vi "Two While Loops.vi"() -> ()   [LabVIEW 2014]
panel:
  out "Bot Variable Stop":bool
  out "Top Variable Stop":bool
  out "Bottom Count":dbl
  in  "stop":bool
  out "Top Count":dbl
  # "Two While Loops"
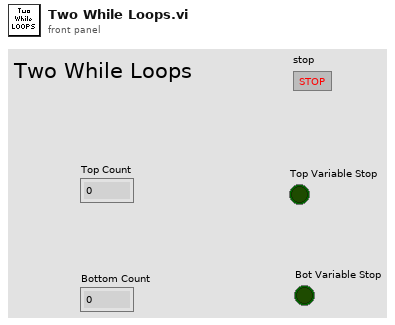
[diagram p1: front panel]
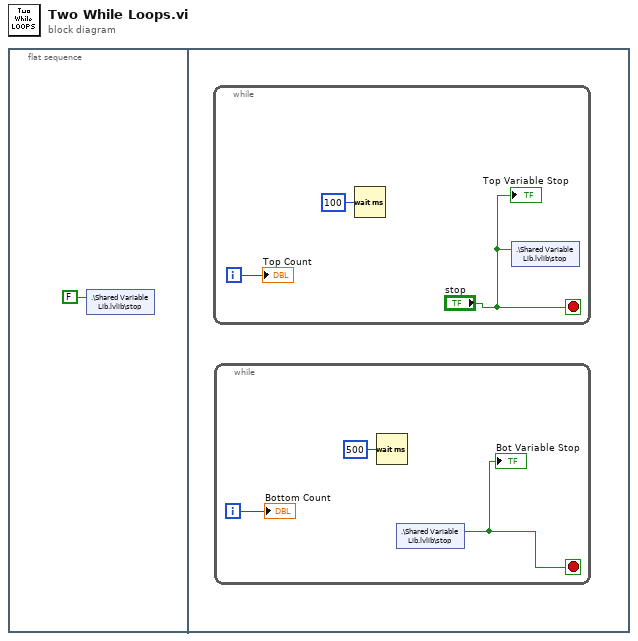
[diagram p0: block diagram]
diagram:
  n1 = flat-sequence {
    frame #0 {
      n2 = shared-variable ".\\Shared Variable Lib.lvlib\\stop"(FALSE ("stop")) -> ()  [unwired: 1 in, 1 out]
    }
    frame #1 {
      n3 = while {
        i -> [w6]
        stop <- "stop" stop-if-true
        n4 = Wait (ms)(milliseconds to wait=u32 100) -> ()  [unwired: 1 out]
        n5 = shared-variable ".\\Shared Variable Lib.lvlib\\stop"("stop") -> ()  [unwired: 1 in, 1 out]
        "Top Count" <- w6
        "Top Variable Stop" <- "stop"
      }
      n6 = while {
        i -> [w4]
        stop <- w2 stop-if-true
        n7 = Wait (ms)(milliseconds to wait=u32 500) -> ()  [unwired: 1 out]
        n8 = shared-variable ".\\Shared Variable Lib.lvlib\\stop"() -> (w2:bool)  [unwired: 1 in, 1 out]
        "Bot Variable Stop" <- w2
        "Bottom Count" <- w4
      }
    }
  }
